vi "Drag Location.vi"(8 "error in (no error)":errorcluster, 9 "Coords":T4, 10 "BetterDropOp":refnum<class "BetterDropOp.lvclass">, 11 "BetterBoxHandle in":refnum<class "BetterBoxHandle.lvclass">) -> (0 "error out":errorcluster, 2 "DragOver Output":T1={"Displayed Row"=0, "Position"=enum."On Row", "Row's TreeItem index"=0, "indent"=0, "Accepted?"=FALSE, "Insertion index"=0, "Top left visible TreeItem index"=0, "Bar type"=enum."tilda up"}, 3 "BetterBoxHandle out":refnum<class "BetterBoxHandle.lvclass">)   [LabVIEW 2020, in "BetterDragAndDrop.lvlib" / "BetterBoxHandle.lvclass"]
uses:
  BetterBoxHandle.lvclass
  BetterDropOp/BetterDropOp.lvclass
  C:/DSCE code/Open-source/betterdraganddrop_GIT/Source/Classes/BetterHandle/BetterHandle.lvclass
  <vilib>/Utility/miscctls.llb/LVPoint32TypeDef.ctl
  SubVIs/DragOver Output.ctl
  SubVIs/DragOverPosition.ctl
  BetterTreeBar/SubVIs/Horizontal Bar Enumeration.ctl
  BetterHandle/BetterHandle.lvclass/BetterHandle.ctl
  BetterHandle/BetterHandle.lvclass
  BetterTreeBar/BetterHorizontalBar.lvclass
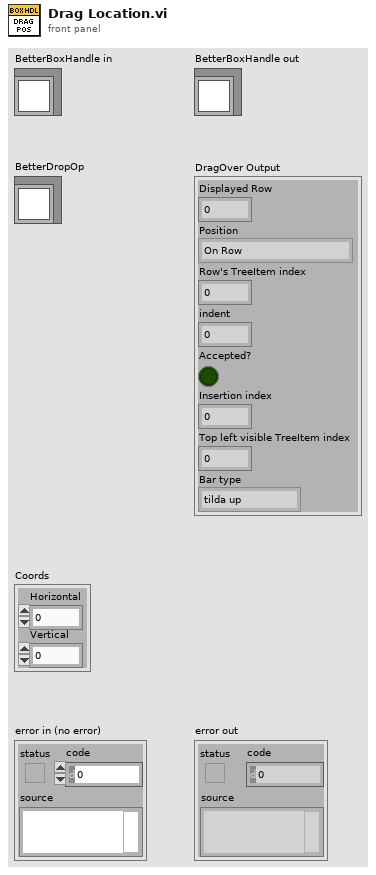
[diagram p1: front panel]
types:
  T1 = typedef "BetterDragAndDrop.lvlib/BetterHandle.lvclass/DragOver Output.ctl" = cluster{"Displayed Row":i32, "Position":T2, "Row's TreeItem index":i32, "indent":i32, "Accepted?":bool, "Insertion index":i32, "Top left visible TreeItem index":i32, "Bar type":T3}
  T2 = typedef "BetterDragAndDrop.lvlib/BetterHandle.lvclass/DragOverPosition.ctl" = enum16{"On Row", "Inbetween"}
  T3 = typedef "BetterDragAndDrop.lvlib/BetterHorizontalBar.lvclass/Horizontal Bar Enumeration.ctl" = enum16{"None", "only bar", "tilda up"}
  T4 = typedef "LVPoint32TypeDef.ctl" = cluster{"Horizontal":i32, "Vertical":i32}
  T5 = typedef "LVPositionTypeDef.ctl" = cluster{"Left":i32, "Top":i32}
  T6 = typedef "BetterDragAndDrop.lvlib/BetterHandle.lvclass/Pixel Constants.ctl" = cluster{"Row Header height":i32, "Row height":i32, "Column Header Offset":i32}
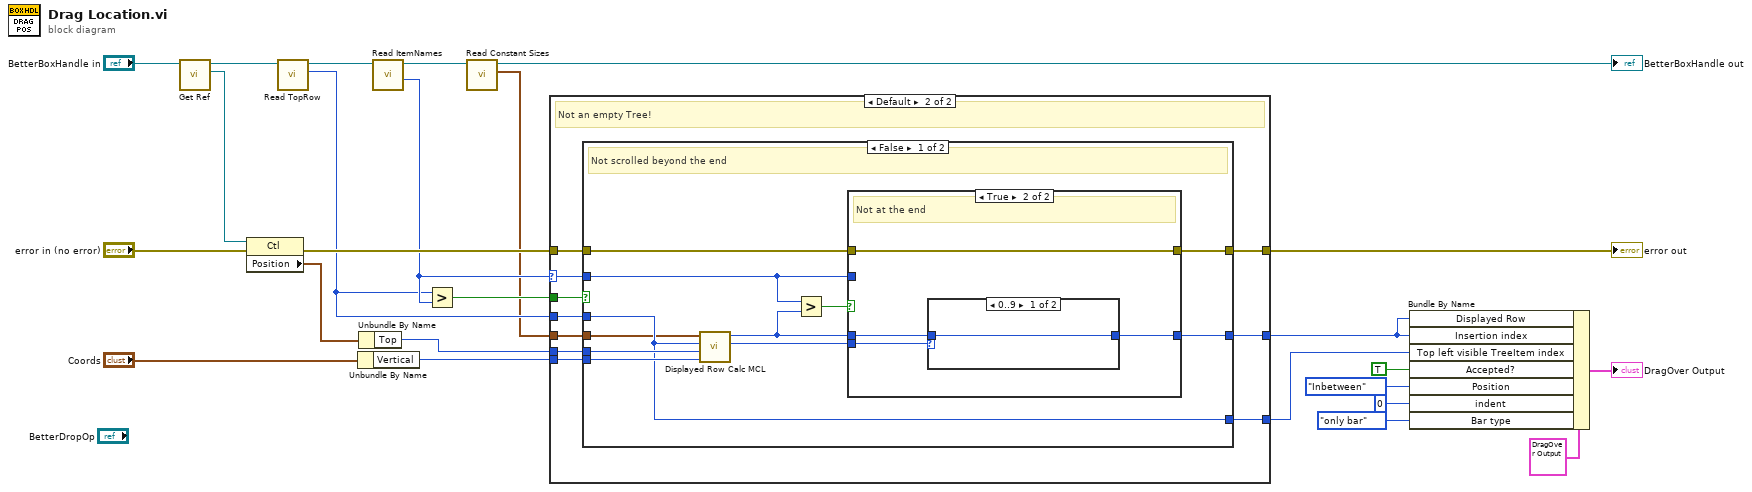
[diagram p0: block diagram]
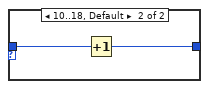
[diagram p4: hidden frame]
diagram:
  n1 = call-dynamic "Get Ref.vi"("BetterHandle in"="BetterBoxHandle in") -> ("Tree/LB/MCL ref"=w16:refnum<vi>, "BetterHandle out"=w19:refnum<class "BetterBoxHandle.lvclass">)  [unwired: 8 in, 1 out]
  n2 = property class="Ctl"(reference=w16, error in="error in (no error)") -> (error out=w23:errorcluster, "Position"=w17:T5)  [unwired: 1 out]
  n3 = call-dynamic "Read TopRow.vi"("BetterBoxHandle in"=w19) -> ("TopRow"=w14:i32, "BetterBoxHandle out"=w18:refnum<class "BetterBoxHandle.lvclass">)  [unwired: 8 in, 1 out]
  n4 = Unbundle By Name("Coords") -> ("Vertical"=w24:i32)
  n5 = Unbundle By Name(w17) -> ("Top"=w22:i32)
  n6 = call-dynamic "Read ItemNames.vi"("BetterBoxHandle in"=w18) -> ("Number of ItemNames"=w15:i32, "BetterBoxHandle out"=w3:refnum<class "BetterBoxHandle.lvclass">)  [unwired: 7 in, 2 out]
  n7 = Greater?(x=w14, y=w15) -> (0:w21:bool)
  n8 = call "Read Constant Sizes.vi"("BetterHandle in"=w3) -> ("constant pixel sizes"=w1:T6, "BetterHandle out"=→"BetterBoxHandle out":refnum<class "BetterBoxHandle.lvclass">)  [unwired: 8 in, 1 out]
  n9 = case shown="Default" w15 {
    selector: w15 -> [_ w34]
    tunnel: w24 -> [_ w31]
    tunnel: [w26 w36] -> w12
    tunnel: w23 -> [w26 w35]
    tunnel: w22 -> [_ w32]
    tunnel: [_ w33] -> w4
    tunnel: w14 -> [_ w30]
    tunnel: w21 -> [_ w29]
    tunnel: [_ w28] -> w10
    tunnel: w1 -> [_ w27]
    frame 0 {
      # "Empty Tree.  This must go at the top"
    }
    frame Default {
      # "Not an empty Tree!"
      n10 = case shown="False" w29 {
        tunnel: [w47 w58] -> w36
        tunnel: w35 -> [w46 w58]
        tunnel: w34 -> [w44 w57]
        tunnel: [w43 w57] -> w33
        tunnel: w32 -> [w42 _]
        tunnel: w31 -> [w41 _]
        tunnel: w30 -> [w38 _]
        tunnel: [w38 w57] -> w28
        tunnel: w27 -> [w37 _]
        frame False {
          # "Not scrolled beyond the end"
          n11 = call "Displayed Row Calc MCL.vi"("Coords.Vertical"=w41, "Tree.Position:Top"=w42, "TopLeft.Row"=w38, "Constant Sizes"=w37) -> ("Pixels from top of row"=w39:i32, "Displayed Row"=w40:i32)  [unwired: 6 in]
          n12 = Greater?(x=w44, y=w40) -> (0:w45:bool)
          n13 = case shown="True" w45 {
            tunnel: w39 -> [_ w53]
            tunnel: [w49 w50] -> w47
            tunnel: w46 -> [w49 w50]
            tunnel: w40 -> [_ w52]
            tunnel: w44 -> [w48 _]
            tunnel: [w48 w51] -> w43
            frame False {
              # "beyond the end"
            }
            frame True {
              # "Not at the end"
              n14 = case shown="0..9" w53 {
                tunnel: w52 -> [w54 w56]
                tunnel: [w54 w55] -> w51
                frame 0..9 {
                }
                frame 10..18, Default {
                  n15 = Increment(x=w56) -> (x+1=w55:i32)
                }
              }
            }
          }
        }
        frame True {
          # "niche case: we are scrolled beyond the end of the tree content"
        }
      }
    }
  }
  "error out" <- w12
  n16 = Bundle By Name(cluster=T1 {"Displayed Row"=0, "Position"=enum."On Row", "Row's TreeItem index"=0, "indent"=0, "Accepted?"=FALSE, "Insertion index"=0, "Top left visible TreeItem index"=0, "Bar type"=enum."tilda up"} ("DragOver Output"), "Displayed Row"=w4, "Insertion index"=w4, "Top left visible TreeItem index"=w10, "Accepted?"=TRUE, "Position"=DragOverPosition."Inbetween", "indent"=0, "Bar type"=Horizontal_Bar_Enumeration."only bar") -> (→"DragOver Output":T1)
